vi "Make Connections (Serial).vi"(8 "error in (no error)":errorcluster, 10 "switchActionsArray":T1 {"RelayAction" items=["CloseRelay"=21, "OpenRelay"=20]}, 11 "SLSC Switch in":refnum<class "SLSC Switch.lvclass">) -> (0 "error out":errorcluster, 3 "SLSC Switch out":refnum<class "SLSC Switch.lvclass">)   [LabVIEW 2015]
uses:
  slscsl/SwitchActionsArray.ctl
  slscsl/SwitchAction.ctl
  slscsl/RelayAction.ctl
  SLSC Switch.lvclass
  Relay Interface/RelayInterface.lvclass
  slscsl/slscsl.lvclass
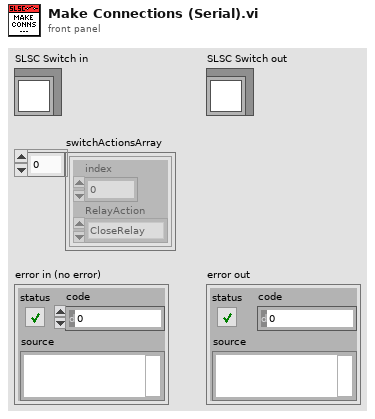
[diagram p1: front panel]
types:
  T1 = typedef "SLSC Switch.lvlib/slscsl.lvclass/SwitchActionsArray.ctl" = T2[]
  T2 = typedef "SLSC Switch.lvlib/slscsl.lvclass/SwitchAction.ctl" = cluster{"index":i32, "RelayAction":T3}
  T3 = typedef "SLSC Switch.lvlib/slscsl.lvclass/RelayAction.ctl" = u32
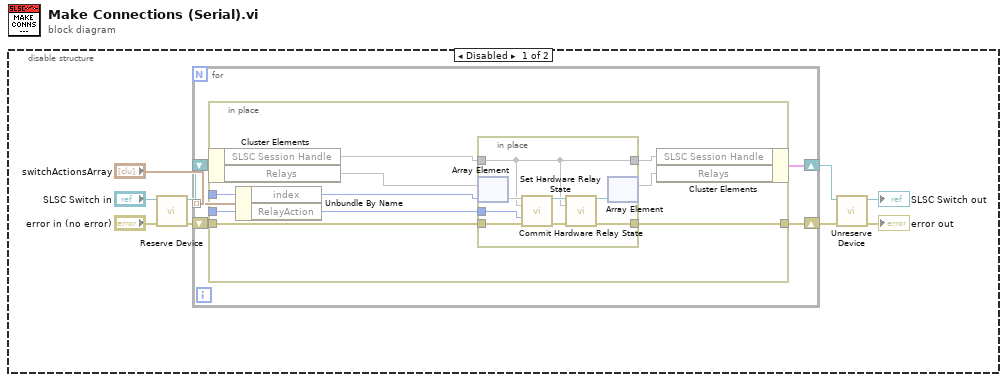
[diagram p0: block diagram]
diagram:
  n1 = disable-structure shown="Disabled" {
    frame Disabled {
      n2 = call "Reserve Device.vi"("error in (no error)"="error in (no error)", "SLSC Switch in"="SLSC Switch in") -> ("error out"=w3:errorcluster, "SLSC Switch out"=w4:refnum<class "SLSC Switch.lvclass">)  [unwired: 8 in]
      n3 = for {
        tunnel: "switchActionsArray" -> [w16] mode=indexing
        shift-right: [w11] -> w2
        shift-left: w4 -> [w13]
        shift-right: [w14] -> w1
        shift-left: w3 -> [w15]
        n4 = Unbundle By Name(w16) -> ("index"=w12:i32, "RelayAction"=w10:T3)
        n5 = in-place {
          in-place-border: w15 -> [w24]
          in-place-border: w10 -> [w23]
          in-place-border: [w22] -> w14
          in-place-border: w12 -> [w20]
          n6 = in-place-cluster #1(w13) -> ("SLSC Session Handle"=w18, "Relays"=w21)
          n7 = in-place {
            in-place-border: w24 -> [w32]
            in-place-border: w23 -> [w31]
            in-place-border: [w26] -> w22
            in-place-border: w18 -> [w25]
            in-place-border: [w25] -> w17
            n8 = in-place-array #2(w21, w20) -> (w30)
            n9 = call-dynamic "Set Hardware Relay State.vi"("RelayInterface in"=w30, "Session Handle in"=w25, "relay action (Close Relay)"=w31, "error in (no error)"=w32) -> ("RelayInterface out"=w29:refnum<class "RelayInterface.lvclass">, "error out"=w27:errorcluster)  [unwired: 10 in]
            n10 = call-dynamic "Commit Hardware Relay State.vi"("RelayInterface in"=w29, "Session Handle in"=w25, "error in (no error)"=w27) -> ("RelayInterface out"=w28:refnum<class "RelayInterface.lvclass">, "error out"=w26:errorcluster)  [unwired: 11 in]
            n11 = in-place-array #2(w28) -> (w19)  [unwired: 1 out]
          }
          n12 = in-place-cluster #1("SLSC Session Handle"=w17, "Relays"=w19) -> (w11:cluster{})
        }
      }
      n13 = call "Unreserve Device.vi"("error in (no error)"=w1, "SLSC Switch in"=w2) -> ("error out"=→"error out":errorcluster, "SLSC Switch out"=→"SLSC Switch out":refnum<class "SLSC Switch.lvclass">)  [unwired: 8 in]
    }
    frame Enabled {
    }
  }
